vi "Drive_Loop_Initialize.vi"(10 "Drive Train Ref":T1={"Sensor Data"={"Gyro Data"={"Gyro RT FIFO"=refnum, "Gyro Current"=0.0, "Gyro Hold"=0.0}, "Encoder Data"={"Encoder RT FIFO"=refnum, "Encoder Current"=0.0, "Encoder Hold"=0.0}, "Camera Data"={"Camera RT FIFO"=refnum, "Camera Current"={" Angle"=0.0, "Valid"=FALSE}}}, "PID Update"=refnum, "RobotDriveDevRef"={"DevStatus"={"status"=FALSE, "code"=0, "source"=""}, "Motors[]"=[], "Square Inputs"=FALSE, "Max Output"=1.0}, "Drive Train"=enum."Tank Drive 2 Motor", "Valid Commands"=[], "Drive Comand Notifier"=refnum}, 11 "Name":string) -> (3 "Drive DevRef Out":T1={"Sensor Data"={"Gyro Data"={"Gyro RT FIFO"=refnum, "Gyro Current"=0.0, "Gyro Hold"=0.0}, "Encoder Data"={"Encoder RT FIFO"=refnum, "Encoder Current"=0.0, "Encoder Hold"=0.0}, "Camera Data"={"Camera RT FIFO"=refnum, "Camera Current"={" Angle"=0.0, "Valid"=FALSE}}}, "PID Update"=refnum, "RobotDriveDevRef"={"DevStatus"={"status"=FALSE, "code"=0, "source"=""}, "Motors[]"=[], "Square Inputs"=FALSE, "Max Output"=1.0}, "Drive Train"=enum."Tank Drive 2 Motor", "Valid Commands"=[], "Drive Comand Notifier"=refnum})   [LabVIEW 2016]
doc: "Help written by FRC Team 836 - The RoboBees\n\nThis VI creates and intializes the RT FIFOs used in the Chessy Drive drive routines."
uses:
  <userlib>/836-libraries/Drive/Drive_Code_V2/Drive_Code_Support/Drive_Code_Bundle.ctl
  <userlib>/836-libraries/Drive/Drive_Code_V2/Drive_Code_Support/SensorTypedefs/Sensor_Cluster.ctl
  <userlib>/836-libraries/Drive/Drive_Code_V2/Drive_Code_Support/SensorTypedefs/Camera_Cluster.ctl
  <userlib>/836-libraries/Drive/Drive_Code_V2/Drive_Code_Support/Drive_Code_PID_Bundle.ctl
  <vilib>/Rock Robotics/WPI/RobotDrive/WPI_RobotDriveDevRef.ctl
  <vilib>/Rock Robotics/WPI/MotorControl/WPI_MotorControlDeviceRef.ctl
  <vilib>/Rock Robotics/WPI/MotorControl/WPI_MotorControlType.ctl
  <vilib>/Rock Robotics/SystemInterfaces/DIO/FPGA_DIOPWMChannel.ctl
  <vilib>/Rock Robotics/WPI/PWM/WPI_PWMDeadband.ctl
  <userlib>/836-libraries/Drive/Drive_Code_V2/Drive_Code_Support/DriveTrains/Drive_Trains.ctl
  <userlib>/836-libraries/Drive/Drive_Code_V2/Drive_Code_Support/Command_Sends/Drive_Code_Command_Type.ctl
  <userlib>/836-libraries/Drive/Drive_Code_V2/Drive_Code_Support/Command_Sends/Drive_Code_Command_List.ctl
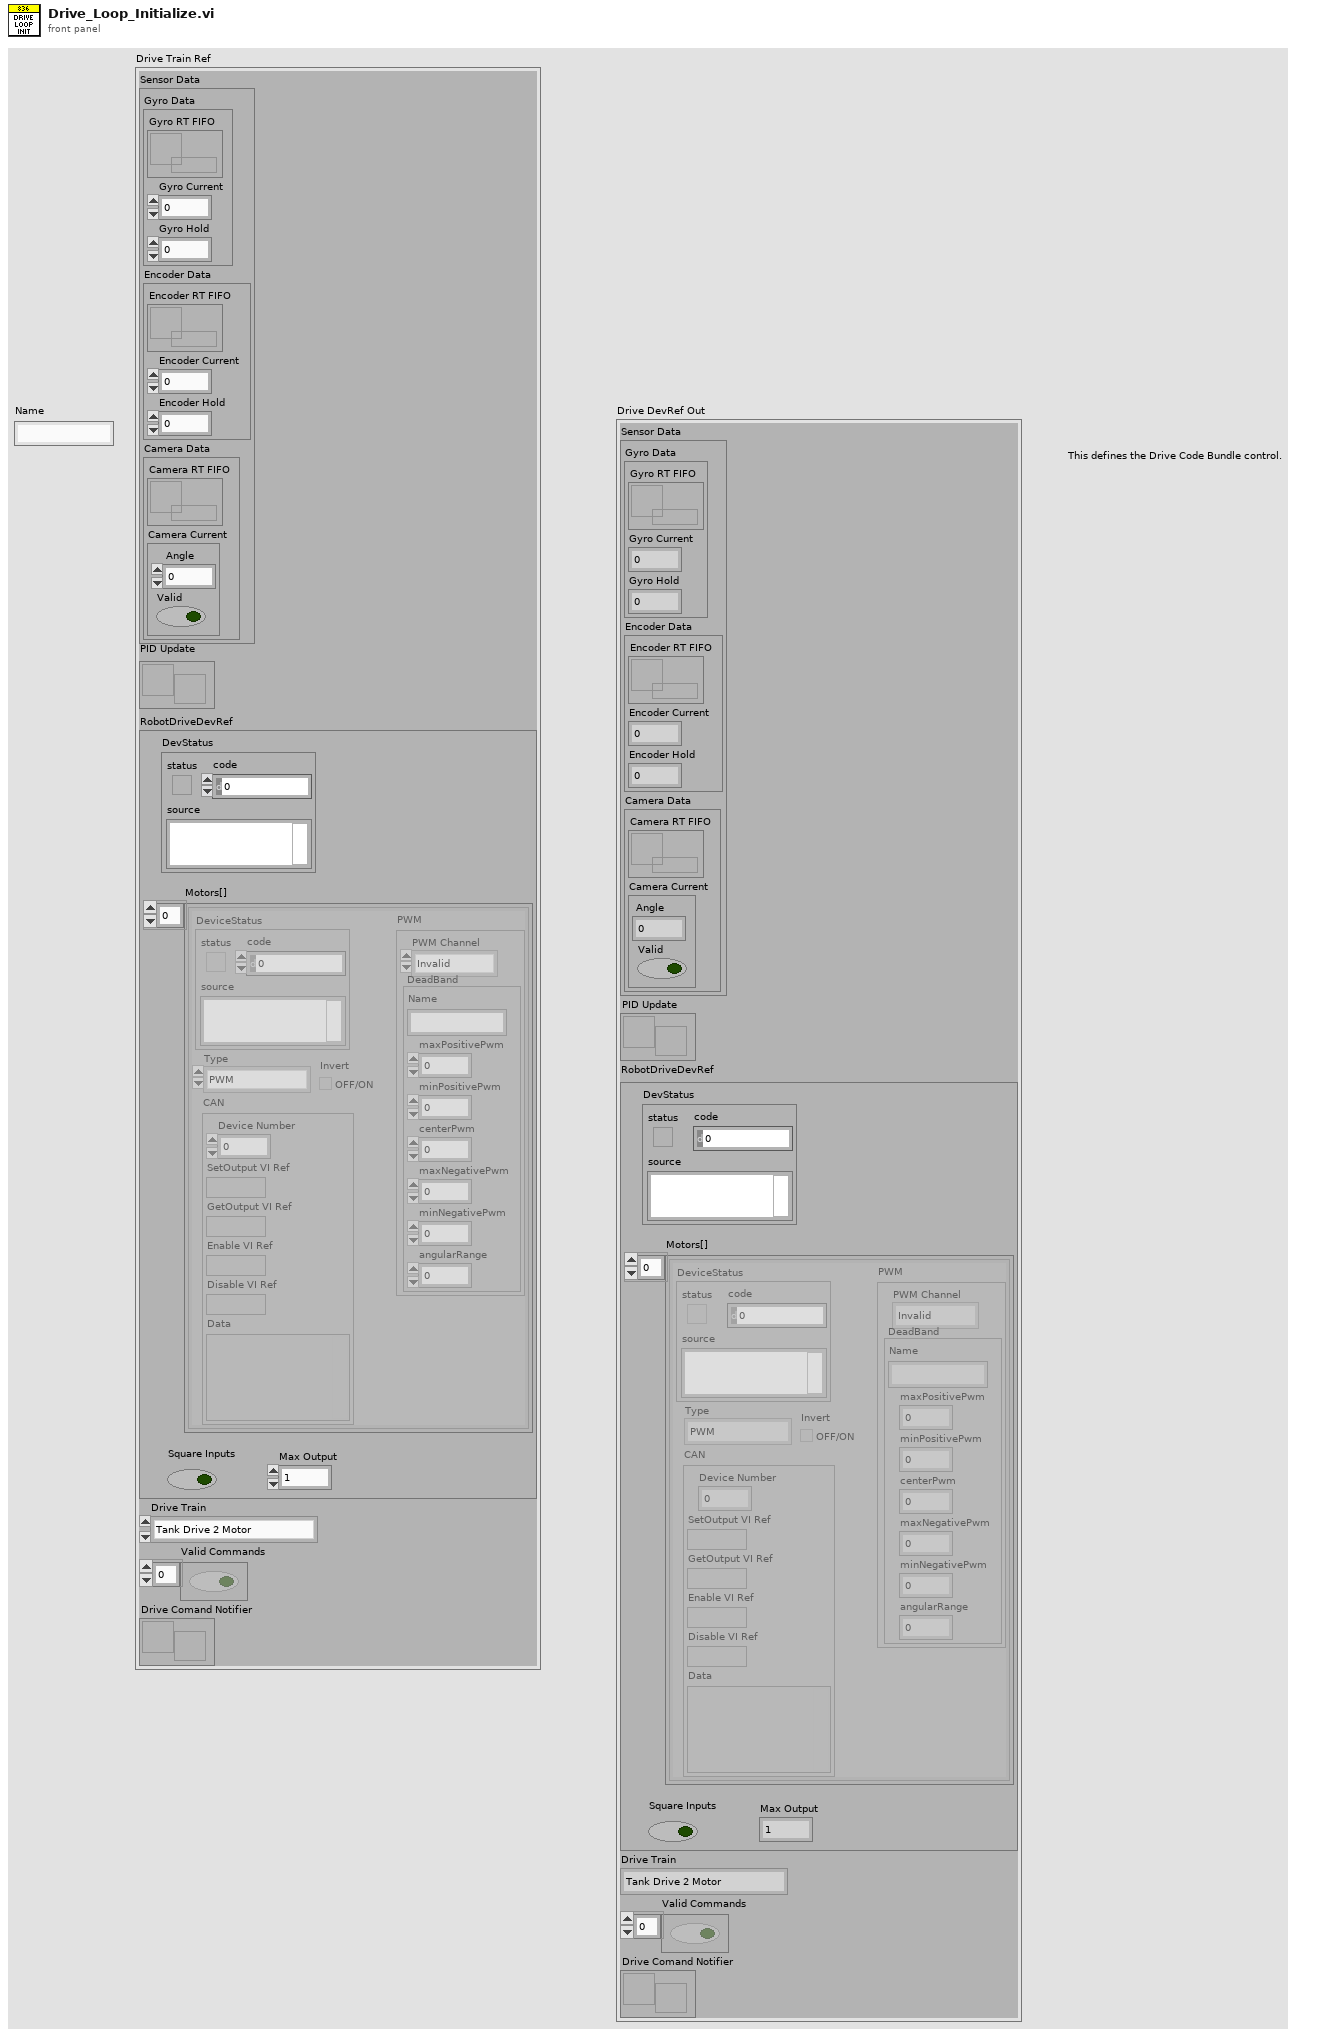
[diagram p1: front panel]
types:
  T1 = typedef "Drive_Code_Bundle.ctl" = cluster{"Sensor Data":T2, "PID Update":refnum<notifier>, "RobotDriveDevRef":T4, "Drive Train":T9, "Valid Commands":bool[], "Drive Comand Notifier":refnum<notifier>}
  T2 = typedef "Sensor_Cluster.ctl" = cluster{"Gyro Data":cluster{"Gyro RT FIFO":refnum<k33>, "Gyro Current":dbl, "Gyro Hold":dbl}, "Encoder Data":cluster{"Encoder RT FIFO":refnum<k33>, "Encoder Current":dbl, "Encoder Hold":dbl}, "Camera Data":cluster{"Camera RT FIFO":refnum<k33>, "Camera Current":T3}}
  T3 = typedef "Camera_Cluster.ctl" = cluster{" Angle":dbl, "Valid":bool}
  T4 = typedef "WPI_RobotDriveDevRef.ctl" = cluster{"DevStatus":errorcluster, "Motors[]":T5[], "Square Inputs":bool, "Max Output":dbl}
  T5 = typedef "WPI_MotorControlDeviceRef.ctl" = cluster{"DeviceStatus":errorcluster, "Type":T6, "PWM":cluster{"PWM Channel":T7, "DeadBand":T8}, "CAN":cluster{"Device Number":u8, "SetOutput VI Ref":variant, "GetOutput VI Ref":variant, "Enable VI Ref":variant, "Disable VI Ref":variant, "Data":variant}, "Invert":bool}
  T6 = typedef "WPI_MotorControlType.ctl" = enum16{"PWM", "CAN"}
  T7 = typedef "FPGA_DIOPWMChannel.ctl" = enum8{"PWM 0", "PWM 1", "PWM 2", "PWM 3", "PWM 4", "PWM 5", "PWM 6", "PWM 7", "PWM 8", "PWM 9", "PWM MXP 0", "PWM MXP 1", "PWM MXP 2", "PWM MXP 3", "PWM MXP 4", "PWM MXP 5", "PWM MXP 6", "PWM MXP 7", "PWM MXP 8", "PWM MXP 9", "Invalid"}
  T8 = typedef "WPI_PWMDeadband.ctl" = cluster{"Name":string, "maxPositivePwm":i32, "minPositivePwm":i32, "centerPwm":i32, "maxNegativePwm":i32, "minNegativePwm":i32, "angularRange":u16}
  T9 = typedef "Drive_Trains.ctl" = enum16{"Tank Drive 2 Motor", "Tank Drive 4 Motor", "Mecanum Drive", "Kiwi Drive"}
  T10 = typedef "Drive_Code_Command_Type.ctl" = cluster{"Command":T11, "Parameter A":dbl, "Parameter B":dbl, "Parameter C":dbl, "Absolute?":bool}
  T11 = typedef "Drive_Code_Command_List.ctl" = enum16{"Do Nothing", "Manual", "Drive Continuous", "Turn", "Drive Distance", "Hold Position", "Hold Yaw", "Follow Camera", "Turn to Camera", "Approach Camera"}
  T12 = typedef "Drive_Code_PID_Bundle.ctl" = cluster{"Yaw, Driving Straight":cluster{"proportional gain (Kc)":dbl, "integral time (Ti, min)":dbl, "derivative time (Td, min)":dbl}, "Yaw, Holding Still":cluster{"proportional gain (Kc)":dbl, "integral time (Ti, min)":dbl, "derivative time (Td, min)":dbl}, "Distance, Driving Straight":cluster{"proportional gain (Kc)":dbl, "integral time (Ti, min)":dbl, "derivative time (Td, min)":dbl}, "Distance, Holding Still":cluster{"proportional gain (Kc)":dbl, "integral time (Ti, min)":dbl, "derivative time (Td, min)":dbl}}
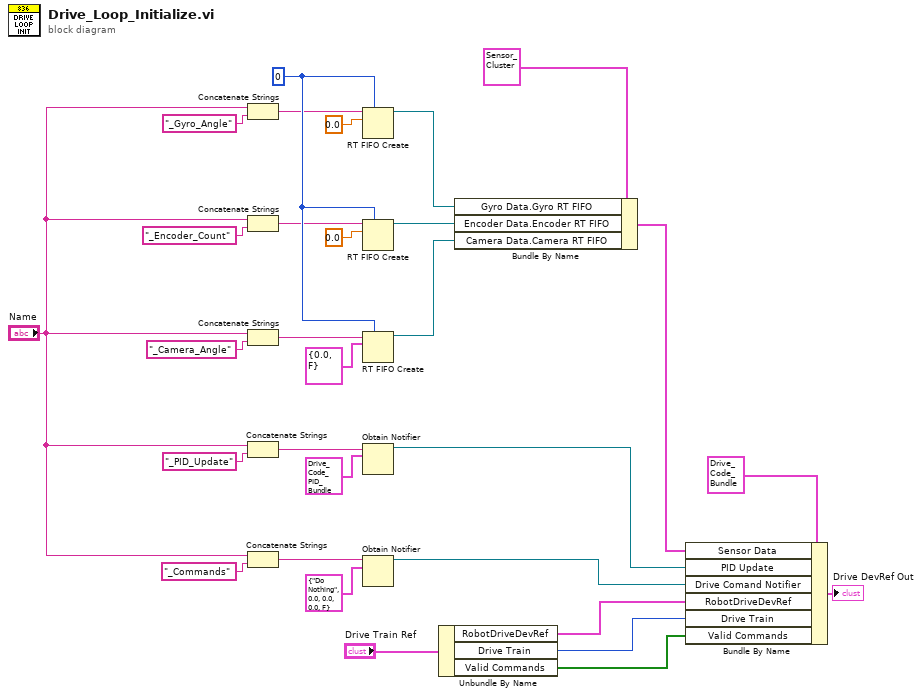
[diagram p0: block diagram]
diagram:
  w27 = u32 0
  n1 = Concatenate Strings("Name", "_Gyro_Angle" ("string")) -> (w24:string)
  n2 = Concatenate Strings("Name", "_Encoder_Count" ("string")) -> (w23:string)
  n3 = Concatenate Strings("Name", "_Camera_Angle" ("string")) -> (w22:string)
  n4 = Concatenate Strings("Name", "_PID_Update" ("string")) -> (w21:string)
  n5 = Concatenate Strings("Name", "_Commands" ("string")) -> (w20:string)
  n6 = RT FIFO Create(0:w24, 1:0.0, 4:w27) -> (8:w11:refnum<k33>)  [unwired: 5 in, 2 out]
  n7 = RT FIFO Create(0:w23, 1:0.0, 4:w27) -> (8:w10:refnum<k33>)  [unwired: 5 in, 2 out]
  n8 = RT FIFO Create(0:w22, 1:T3 {" Angle"=0.0, "Valid"=FALSE} ("Cluster"), 4:w27) -> (8:w9:refnum<k33>)  [unwired: 5 in, 2 out]
  n9 = Obtain Notifier(name (unnamed)=w21, notification data type=T12 {"Yaw, Driving Straight"={"proportional gain (Kc)"=1.0, "integral time (Ti, min)"=0.01, "derivative time (Td, min)"=0.0}, "Yaw, Holding Still"={"proportional gain (Kc)"=1.0, "integral time (Ti, min)"=0.01, "derivative time (Td, min)"=0.0}, "Distance, Driving Straight"={"proportional gain (Kc)"=1.0, "integral time (Ti, min)"=0.01, "derivative time (Td, min)"=0.0}, "Distance, Holding Still"={"proportional gain (Kc)"=1.0, "integral time (Ti, min)"=0.01, "derivative time (Td, min)"=0.0}} ("PID Gains")) -> (notifier out=w7:refnum<notifier>)  [unwired: 2 in, 2 out]
  n10 = Obtain Notifier(name (unnamed)=w20, notification data type=T10 {"Command"=enum."Do Nothing", "Parameter A"=0.0, "Parameter B"=0.0, "Parameter C"=0.0, "Absolute?"=FALSE} ("Cluster")) -> (notifier out=w6:refnum<notifier>)  [unwired: 2 in, 2 out]
  n11 = Unbundle By Name("Drive Train Ref") -> ("RobotDriveDevRef"=w4:T4, "Drive Train"=w3:T9, "Valid Commands"=w2:bool[])
  n12 = Bundle By Name(cluster=T2 {"Gyro Data"={"Gyro RT FIFO"=refnum, "Gyro Current"=0.0, "Gyro Hold"=0.0}, "Encoder Data"={"Encoder RT FIFO"=refnum, "Encoder Current"=0.0, "Encoder Hold"=0.0}, "Camera Data"={"Camera RT FIFO"=refnum, "Camera Current"={" Angle"=0.0, "Valid"=FALSE}}} ("Cluster"), "Gyro Data.Gyro RT FIFO"=w11, "Encoder Data.Encoder RT FIFO"=w10, "Camera Data.Camera RT FIFO"=w9) -> (w8:T2)
  n13 = Bundle By Name(cluster=T1 {"Sensor Data"={"Gyro Data"={"Gyro RT FIFO"=refnum, "Gyro Current"=0.0, "Gyro Hold"=0.0}, "Encoder Data"={"Encoder RT FIFO"=refnum, "Encoder Current"=0.0, "Encoder Hold"=0.0}, "Camera Data"={"Camera RT FIFO"=refnum, "Camera Current"={" Angle"=0.0, "Valid"=FALSE}}}, "PID Update"=refnum, "RobotDriveDevRef"={"DevStatus"={"status"=FALSE, "code"=0, "source"=""}, "Motors[]"=[], "Square Inputs"=FALSE, "Max Output"=1.0}, "Drive Train"=enum."Tank Drive 2 Motor", "Valid Commands"=[], "Drive Comand Notifier"=refnum} ("Cluster"), "Sensor Data"=w8, "PID Update"=w7, "Drive Comand Notifier"=w6, "RobotDriveDevRef"=w4, "Drive Train"=w3, "Valid Commands"=w2) -> (→"Drive DevRef Out":T1)
